vi "多通道并行实测.vi"() -> ()   [LabVIEW 2020]
uses:
  <vilib>/Utility/sysdir.llb/System Directory Type.ctl
  <vilib>/Utility/error.llb/DialogType.ctl
  global/GlobalVariable.vi
  global/SettingVariable.vi
  <vilib>/Analysis/polynomials.llb/Scalar Polynomial Evaluation (DBL).vi
  <vilib>/Analysis/NI_AALPro.lvlib
panel:
  out "T2周期":dbl[](array[numeric]) caption="倍增周期 (s):"
  in  "拟合数":i32(knob)=5 scale=5.0..100.0
  out "多通道并行测量":dbl[][](graph) caption="Waveform Chart - Dark"
  out "四路VO":dbl[](array[numeric]) caption="四路电压输出(V)："
  out "反应性OUT":dbl[](array[numeric])
  out "源与本底开":bool
  in  "源与本底":bool
  out "滤波开":bool
  in  "通量滤波":bool
  out "DRWM开":bool
  in  "动态刻棒":bool
  in  "全量程衔接设置":bool
  in  "添加备注说明":string caption="添加备注说明："
  in  "Start Button":bool
  in  "停止测量":bool
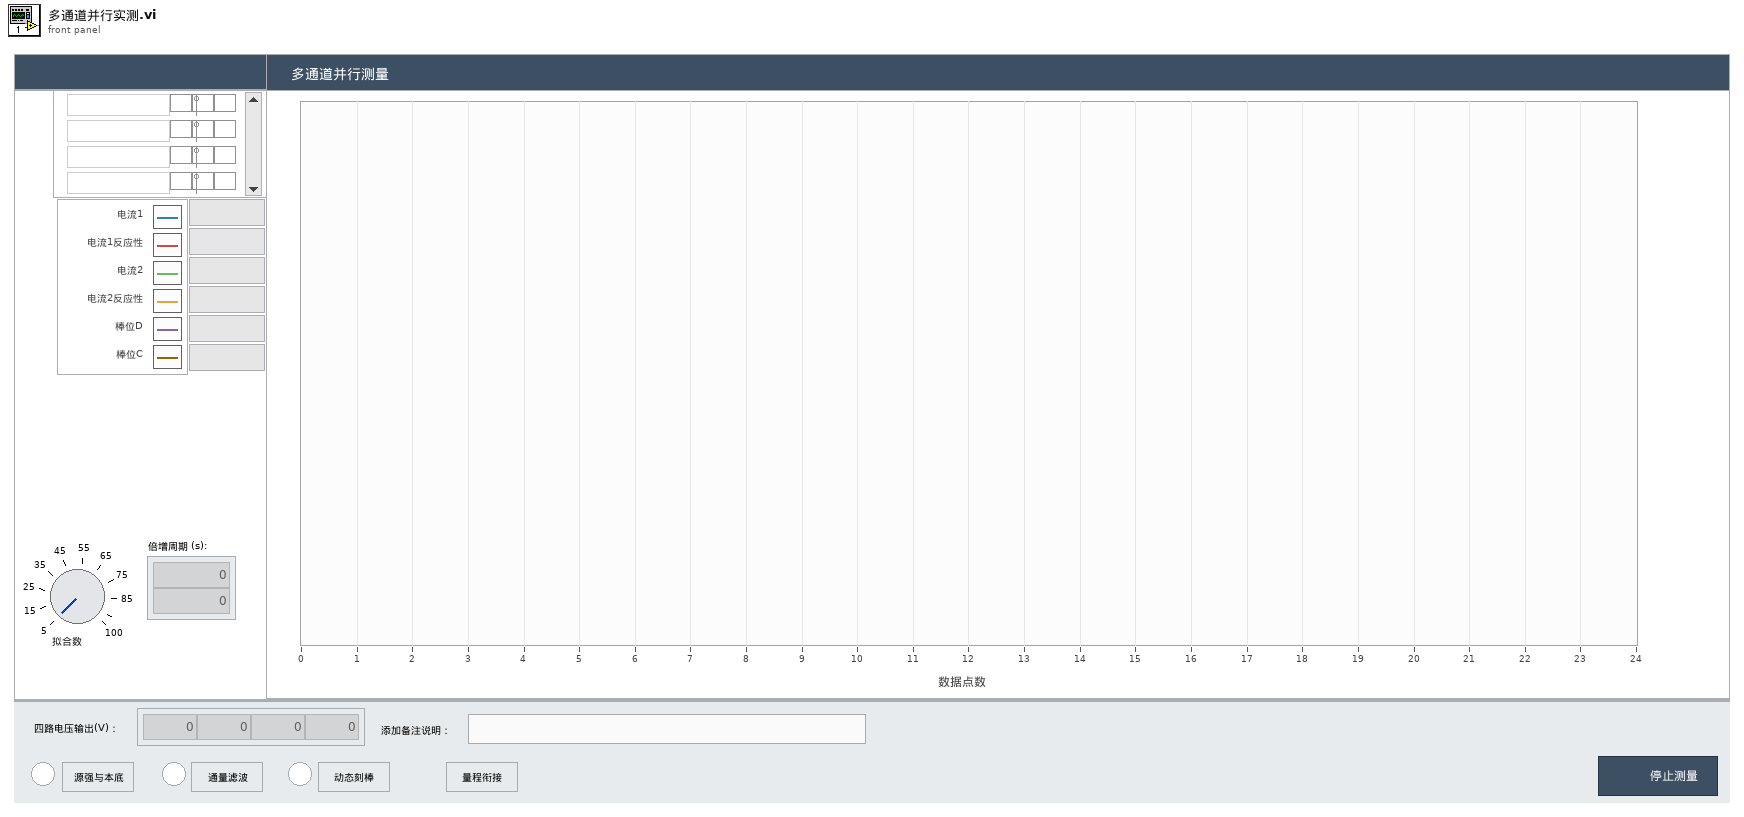
[diagram p1: front panel]
types:
  T1 = enum8{"Enabled", "Disabled", "Disabled and Grayed Out"}
  T2 = enum16{"open", "open or create", "create or replace", "create", "open (read only)"}
  T3 = cluster{"switch":bool, "name":string, "voltage upper":i32, "voltage lower":i32, "physics upper":dbl, "physics lower":dbl, "scale":u16}[]
  T4 = typedef "DialogType.ctl" = u16
  T5 = typedef "System Directory Type.ctl" = i32
  T6 = cluster{"switch":bool, "voltage upper":i32, "voltage lower":i32, "physics upper":dbl, "physics lower":dbl, "input":u16, "log":bool}[]
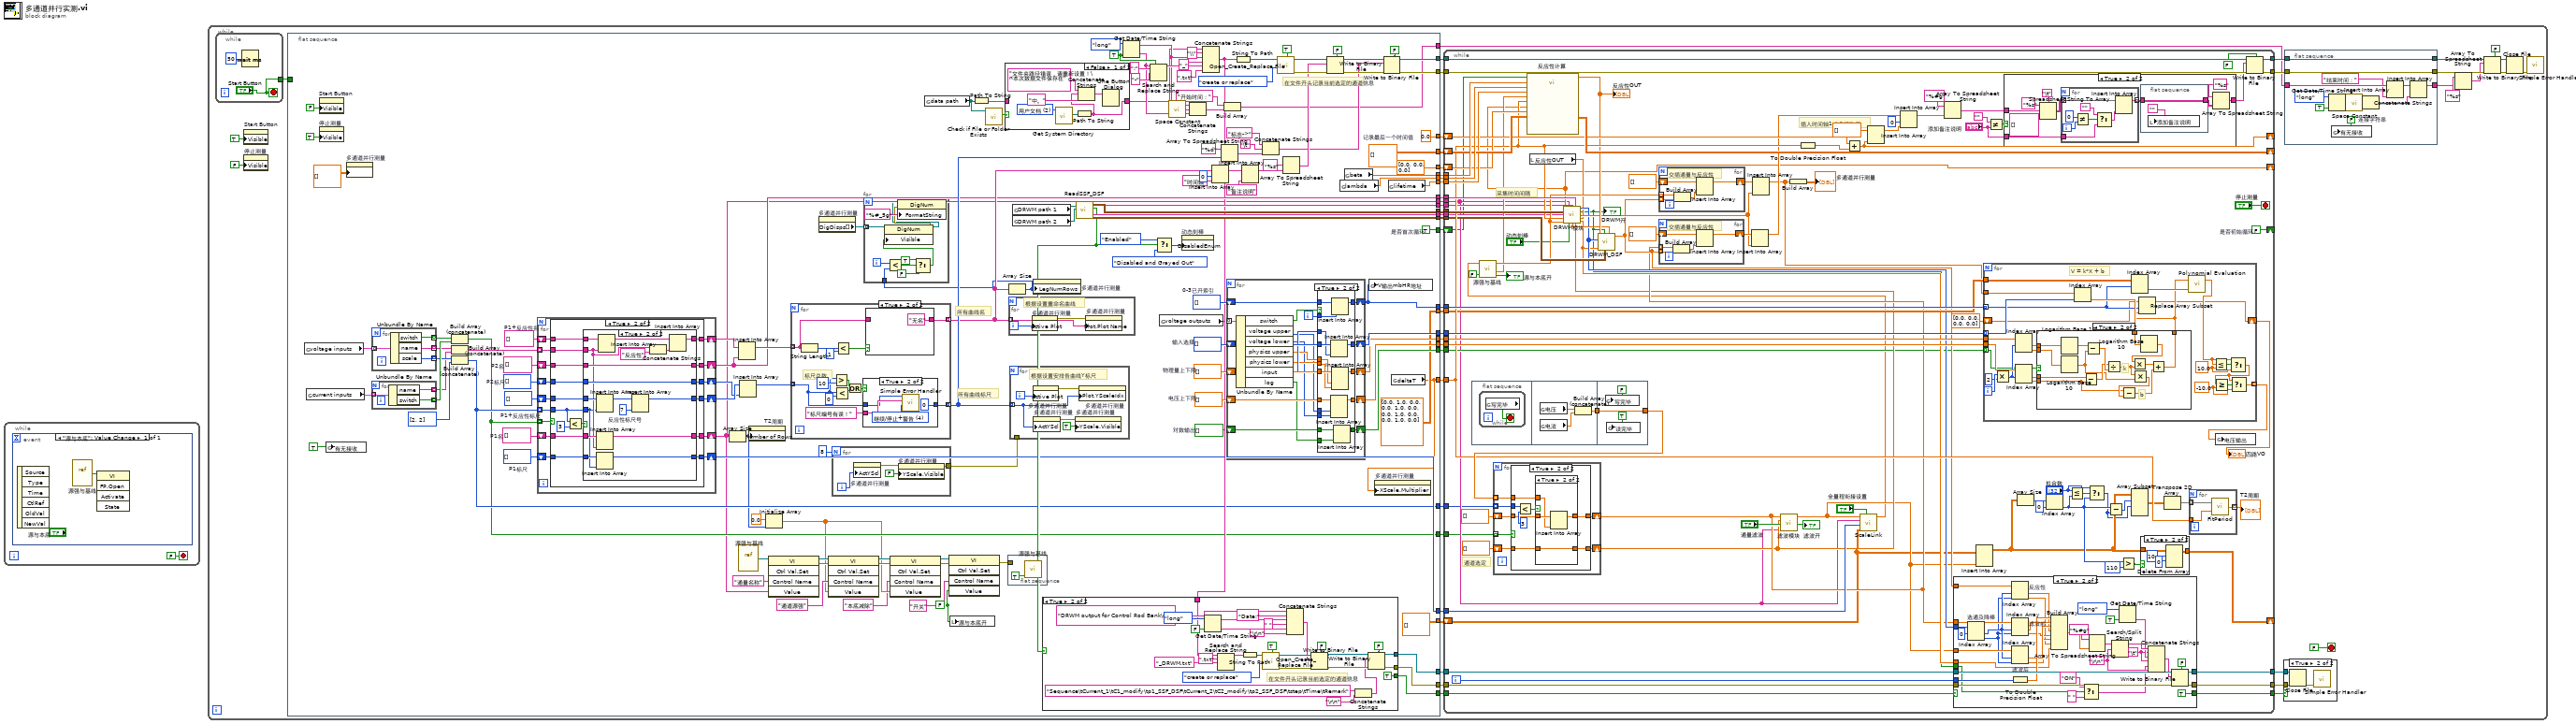
[diagram p0: block diagram]
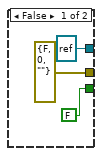
[diagram p4: hidden frame]
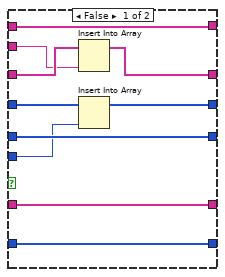
[diagram p8: hidden frame]
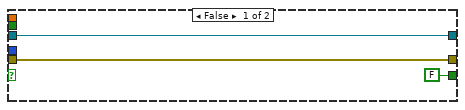
[diagram p10: hidden frame]
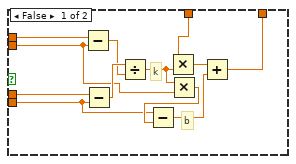
[diagram p12: hidden frame]
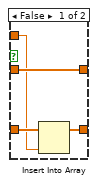
[diagram p15: hidden frame]
diagram:
  n1 = while {
    stop <- FALSE stop-if-true
    n2 = event shown="[0] \"源与本底\": Value Change" {
      selector: _ -> [_]
      dyn-events: _ -> [_]
      timeout: _ -> [_]
      event "源与本底": Value Change {
        n3 = event-data() -> ()  [unwired: 1 in, 6 out]
        n4 = vi-ref "源强与基线.vi"() -> (w2:refnum<vi>)
        n5 = invoke class="VI" method="FP.Open"(reference=w2) -> ()  [unwired: 4 in, 5 out]
      }
    }
  }
  n6 = while {
    stop <- FALSE stop-if-true
    n7 = while {
      tunnel: ["Start Button"] -> w5
      stop <- "Start Button" stop-if-true
      n8 = Wait (ms)(milliseconds to wait=u32 50) -> ()  [unwired: 1 out]
    }
    n9 = property on="Start Button" class="Bool"("Visible"=TRUE) -> ()  [unwired: 2 in, 2 out]
    n10 = property on="停止测量" class="Bool"("Visible"=FALSE) -> ()  [unwired: 2 in, 2 out]
    n11 = flat-sequence {
      tunnel: [sgl[][] [] ("λ*Ci")] -> w50
      tunnel: [w167] -> w47
      tunnel: [w150] -> w46
      tunnel: [w149] -> w45
      tunnel: [w143] -> w44
      tunnel: [sgl[] [0.0, 0.0, 0.0] ("N(0)OUT")] -> w34
      tunnel: [w128] -> w33
      tunnel: [w127] -> w32
      tunnel: [w126] -> w31
      tunnel: [dbl[][] [] ("data")] -> w30
      tunnel: [w122] -> w29
      tunnel: [w114] -> w28
      tunnel: [w113] -> w27
      tunnel: [w112] -> w26
      tunnel: [w111] -> w25
      tunnel: [w110] -> w24
      tunnel: [w109] -> w23
      tunnel: [w107] -> w20
      tunnel: [w104] -> w18
      tunnel: [w103] -> w17
      tunnel: [w102] -> w16
      tunnel: [w101] -> w15
      tunnel: [w98] -> w14
      tunnel: [w67] -> w13
      tunnel: [w86] -> w12
      tunnel: [w85] -> w11
      tunnel: [w84] -> w10
      tunnel: [w72] -> w9
      tunnel: [dbl[][] [[0.0, 1.0, 0.0], [0.0, 1.0, 0.0], [0.0, 1.0, 0.0], [0.0, 1.0, 0.0]]] -> w8
      tunnel: [w78] -> w7
      tunnel: w5 -> [_]
      frame #0 {
        w54 = FALSE
        w87 = i32[] []  # P1标尺
        w88 = string[] []  # P1名
        w105 = bool[] []  # 对数输出
        w124 = i32[] []  # 0-3已开索引
        w129 = sgl[] []  # 电压上下限
        w130 = sgl[] []  # 物理量上下限
        w131 = u16[] []  # 输入选择
        w138 = TRUE ("需要秒？(F)")
        w143 = 0.0  # 记录最后一个时间值
        w163 = string[] []  # P2名
        w162 = i32[] []  # P2标尺
        w164 = i32[] []  # P1+反应性标尺
        w165 = string[] []  # P1+反应性名
        w167 = TRUE  # 是否首次循环
        # "所有曲线标尺"
        # "所有曲线名"
        # "在文件开头记录当前选定的通道信息"
        n12 = global read "SettingVariable.vi" "voltage inputs"() -> (w97:T3)
        n13 = global read "SettingVariable.vi" "current inputs"() -> (w96:cluster{"name":string, "switch":bool}[])
        n14 = property on="Start Button" class="Bool"("Visible"=FALSE) -> ()  [unwired: 2 in, 2 out]
        n15 = property on="停止测量" class="Bool"("Visible"=TRUE) -> ()  [unwired: 2 in, 2 out]
        n16 = global write "GlobalVariable.vi" "有无接收"(TRUE ("写完毕")) -> ()
        n17 = property on="多通道并行测量" class="WFChart (strict)"("History Data"=dbl[][] []) -> ()  [unwired: 2 in, 2 out]
        n18 = for {
          tunnel: w96 -> [w217] mode=indexing
          tunnel: [w216] -> w91 mode=indexing
          tunnel: [w215] -> w94 mode=indexing
          n19 = Unbundle By Name(w217) -> ("name"=w216:string, "switch"=w215:bool)
        }
        n20 = for {
          tunnel: w97 -> [w221] mode=indexing
          tunnel: [w220] -> w95 mode=indexing
          tunnel: [w219] -> w93 mode=indexing
          tunnel: [w218] -> w92 mode=indexing
          n21 = Unbundle By Name(w221) -> ("switch"=w220:bool, "name"=w219:string, "scale"=w218:u16)
        }
        n22 = Build Array (concatenate)(w95, w94) -> (w84:bool[])
        n23 = Build Array (concatenate)(w93, w91) -> (w89:string[])
        n24 = Build Array (concatenate)(w92, u16[] [2, 2] ("array")) -> (w85:u16[])
        n25 = for {
          tunnel: w89 -> [w315] mode=indexing
          shift-right: [w323] -> w161
          shift-left: w165 -> [w322]
          shift-right: [w320] -> w160
          shift-left: w164 -> [w321]
          shift-right: [w318] -> w122
          shift-left: w163 -> [w319]
          shift-right: [w316] -> w159
          shift-left: w162 -> [w317]
          tunnel: w84 -> [w314] mode=indexing
          tunnel: w85 -> [w313] mode=indexing
          shift-right: [w311] -> w67
          shift-left: w88 -> [w312]
          shift-right: [w309] -> w86
          shift-left: w87 -> [w310]
          n26 = case shown="True" w314 {
            tunnel: [w329 w345] -> w323
            tunnel: w322 -> [w329 w341]
            tunnel: w315 -> [_ w340]
            tunnel: [w328 w343] -> w320
            tunnel: w321 -> [w328 w335]
            tunnel: w319 -> [w327 w339]
            tunnel: [w327 w338] -> w318
            tunnel: w317 -> [w326 w337]
            tunnel: [w326 w336] -> w316
            tunnel: w313 -> [_ w334]
            tunnel: w312 -> [w325 w333]
            tunnel: [w325 w332] -> w311
            tunnel: w310 -> [w324 w331]
            tunnel: [w324 w330] -> w309
            frame False {
            }
            frame True {
              n27 = Less?(x=w334, y=3) -> (x < y?=w342:bool)
              n28 = case shown="True" w342 {
                tunnel: w341 -> [w354 w367]
                tunnel: [w354 w372] -> w345
                tunnel: w335 -> [w355 w363]
                tunnel: [w355 w371] -> w343
                tunnel: w340 -> [w351 w360]
                tunnel: w339 -> [w353 w365]
                tunnel: [w352 w365] -> w338
                tunnel: [w348 w364] -> w336
                tunnel: w337 -> [w350 w364]
                tunnel: w334 -> [w349 w356]
                tunnel: w333 -> [w347 w361]
                tunnel: [w347 w359] -> w332
                tunnel: w331 -> [w346 w358]
                tunnel: [w346 w357] -> w330
                frame False {
                  n29 = Insert Into Array(array=w353, new element=w351) -> (w352:string[])  [unwired: 1 in]
                  n30 = Insert Into Array(array=w350, new element=w349) -> (w348:i32[])  [unwired: 1 in]
                }
                frame True {
                  w368 = 7  # 反应性标尺号
                  n31 = Insert Into Array(array=w363, new element=w356) -> (w362:i32[])  [unwired: 1 in]
                  n32 = Insert Into Array(array=w361, new element=w360) -> (w359:string[])  [unwired: 1 in]
                  n33 = Insert Into Array(array=w358, new element=w356) -> (w357:i32[])  [unwired: 1 in]
                  n34 = Insert Into Array(array=w367, new element=w360) -> (w366:string[])  [unwired: 1 in]
                  n35 = Insert Into Array(array=w362, new element=w368) -> (w371:i32[])  [unwired: 1 in]
                  n36 = Concatenate Strings(w360, "反应性" ("字符串")) -> (w369:string)
                  n37 = Insert Into Array(array=w366, new element=w369) -> (w372:string[])  [unwired: 1 in]
                }
              }
            }
          }
        }
        n38 = Array Size(array=w67) -> (size(s)=w66:i32)
        n39 = Insert Into Array(array=w161, new element=w122) -> (w157:string[])  [unwired: 1 in]
        n40 = vi-ref "源强与基线.vi"() -> (w69:refnum<vi>)
        n41 = Insert Into Array(array=w160, new element=w159) -> (w158:i32[])  [unwired: 1 in]
        n42 = property on="T2周期" class="Arr (strict)"("Number of Rows"=w66) -> ()  [unwired: 2 in, 2 out]
        n43 = Initialize Array(0.0 ("element"), w66) -> (w59:dbl[])
        n44 = invoke class="VI" method="Ctrl Val.Set"(reference=w69, "Control Name"="通量名称", "Value"=w67) -> (reference out=w64:refnum<vi>, error out=w63:errorcluster)  [unwired: 2 in, 3 out]
        n45 = for {
          tunnel: w158 -> [w200] mode=indexing
          tunnel: w157 -> [w197] mode=indexing
          tunnel: [w198] -> w148 mode=indexing
          tunnel: [w196] -> w123 mode=indexing
          # "标尺总数"
          n46 = String Length(string=w197) -> (length=w202:i32)
          n47 = Greater?(x=w200, y=10) -> (0:w204:bool)
          n48 = Less?(x=w200, y=0) -> (x < y?=w203:bool)
          n49 = Less?(x=w202, y=1) -> (x < y?=w195:bool)
          n50 = Or(x=w204, y=w203) -> (x .or. y?=w201:bool)
          n51 = case shown="True" w201 {
            tunnel: "标尺编号有误！" ("error source (\" \")") -> [_ w212]
            tunnel: w200 -> [w208 w211]
            tunnel: [w208 0] -> w198
            frame False {
            }
            frame True {
              w210 = T4 4 items=["无对话框", "确定信息", "继续或停止信息", "确定信息＋警告", "继续/停止+警告"] ("type of dialog (OK msg:1)")
              n52 = call <vilib>:"Simple Error Handler.vi"("error code (no error:0)"=w211, "error source (\" \")"=w212, "type of dialog (OK msg:1)"=w210) -> ()  [unwired: 2 in, 5 out]
            }
          }
          n53 = case shown="True" w195 {
            tunnel: w197 -> [w213 _]
            tunnel: [w213 "无名"] -> w196
            frame False {
            }
            frame True {
            }
          }
        }
        n54 = property on="多通道并行测量" class="WFChart (strict)"() -> ("DigDisps[]"=w75:refnum<vi>[])  [unwired: 2 in, 2 out]
        n55 = invoke class="VI" method="Ctrl Val.Set"(reference=w64, error in=w63, "Control Name"="通道源强", "Value"=w59) -> (reference out=w61:refnum<vi>, error out=w60:errorcluster)  [unwired: 1 in, 3 out]
        n56 = for {
          N: 8 -> [_]
          tunnel: [w182] -> w70
          i -> [w181]
          n57 = property on="多通道并行测量" class="WFChart (strict)"("ActYScl"=w181) -> (error out=w183:errorcluster)  [unwired: 2 in, 1 out]
          n58 = property on="多通道并行测量" class="WFChart (strict)"(error in=w183, "YScale.Visible"=FALSE ("Y Scale.Visible")) -> (error out=w182:errorcluster)  [unwired: 1 in, 1 out]
        }
        n59 = invoke class="VI" method="Ctrl Val.Set"(reference=w61, error in=w60, "Control Name"="本底减除", "Value"=w59) -> (reference out=w57:refnum<vi>, error out=w56:errorcluster)  [unwired: 1 in, 3 out]
        n60 = global read "SettingVariable.vi" "data path"() -> (w99:path)
        n61 = invoke class="VI" method="Ctrl Val.Set"(reference=w57, error in=w56, "Control Name"="开关", "Value"=w54) -> (error out=w53:errorcluster)  [unwired: 1 in, 4 out]
        n62 = local write "源与本底开"(w54) -> ()
        n63 = Path To String(path=w99) -> (string=w100:string)
        n64 = call <vilib>:"Check if File or Folder Exists.vi"("path"=w99) -> ("file or folder exists?"=w119:bool)  [unwired: 8 in, 2 out]
        n65 = case shown="False" w119 {
          tunnel: w100 -> [_ w267]
          tunnel: [w262 w267] -> w118
          frame False {
            w266 = T5 2 items=["用户目录"=0, "用户桌面"=1, "用户文档"=2, "用户应用程序数据"=3, "用户设置"=4, "用户临时目录"=5, "公共文档"=6, "公共应用程序数据"=7, "公共设置"=8, "公共缓存"=13, "系统核心库"=9, "系统安装库"=10, "应用程序文件"=11, "启动盘根目录"=12] ("system directory type")
            n66 = call <vilib>:"Get System Directory.vi"("system directory type"=w266) -> ("system directory"=w264:path)  [unwired: 10 in]
            n67 = Path To String(path=w264) -> (string=w262:string)
            n68 = Concatenate Strings("文件夹路径错误，请重新设置！\n本次数据文件保存在" ("消息"), w262, "中。" ("字符串")) -> (w265:string)
            n69 = One Button Dialog(message=w265) -> ()  [unwired: 1 in, 1 out]
          }
          frame True {
          }
        }
        n70 = flat-sequence {
          tunnel: w53 -> [_]
          frame #0 {
            n71 = call "源强与基线.vi"("首次调用？"=TRUE) -> ()  [unwired: 6 in, 3 out]
          }
        }
        n72 = for {
          tunnel: w123 -> [w228] mode=indexing
          i -> [w229]
          # "根据设置重命名曲线"
          n73 = property on="多通道并行测量" class="WFChart (strict)"("Active Plot"=w229) -> (error out=w227:errorcluster)  [unwired: 2 in, 1 out]
          n74 = property on="多通道并行测量" class="WFChart (strict)"(error in=w227, "Plot.Plot Name"=w228) -> ()  [unwired: 1 in, 2 out]
        }
        n75 = Array Size(array=w123) -> (size(s)=w74:i32)
        n76 = for {
          tunnel: w75 -> [w194] mode=indexing
          tunnel: w74 -> [w190]
          i -> [w192]
          n77 = Less?(x=w192, y=w190) -> (x < y?=w191:bool)
          n78 = Select(t=TRUE ("Visible"), s=w191, f=FALSE) -> (s? t:f=w188:bool)
          n79 = property class="DigNum"(reference=w194, "Visible"=w188) -> (reference out=w185:refnum<vi>, error out=w186:errorcluster)  [unwired: 1 in]
          n80 = property class="DigNum"(reference=w185, error in=w186, "FormatString"="%#_5g" ("Format String")) -> ()  [unwired: 2 out]
        }
        n81 = for {
          tunnel: w148 -> [w224] mode=indexing
          tunnel: w70 -> [_]
          i -> [w226]
          # "根据设置安排各曲线Y标尺"
          n82 = property on="多通道并行测量" class="WFChart (strict)"("Active Plot"=w226) -> (error out=w225:errorcluster)  [unwired: 2 in, 1 out]
          n83 = property on="多通道并行测量" class="WFChart (strict)"("ActYScl"=w224) -> (error out=w223:errorcluster)  [unwired: 2 in, 1 out]
          n84 = property on="多通道并行测量" class="WFChart (strict)"(error in=w223, "YScale.Visible"=TRUE ("Y Scale.Visible")) -> ()  [unwired: 1 in, 2 out]
          n85 = property on="多通道并行测量" class="WFChart (strict)"(error in=w225, "Plot.YScaleIdx"=w224) -> ()  [unwired: 1 in, 2 out]
        }
        n86 = global read "SettingVariable.vi" "DRWM path 1"() -> (w80:path)
        n87 = global read "SettingVariable.vi" "DRWM path 2"() -> (w79:path)
        n88 = property on="多通道并行测量" class="WFChart (strict)"("LegNumRows"=w74) -> ()  [unwired: 2 in, 2 out]
        n89 = call "ReadSSF_DSF.vi"("DRWM path 2"=w79, "DRWM path 1"=w80) -> ("DSF"=w113:cluster{"x":dbl, "y":dbl}[][], "因子棒号"=w112:string[], "SF_0K"=w106:bool, "SSF"=w114:cluster{"x":dbl, "y":dbl}[][], "文件INFO"=w111:string)  [unwired: 5 in]
        n90 = Get Date/Time String(date format (0)=enum16{"short", "long", "abbreviated"}."long" ("日期格式(0)"), want seconds? (F)=w138) -> (date string=w136:string, time string=w135:string)  [unwired: 1 in]
        n91 = Search and Replace String(replace all?=w138, input string=w135, search string=":", replace string="-" ("replace string (\"\")")) -> (result string=w174:string)  [unwired: 4 in, 3 out]
        n92 = Select(t=T1."Enabled" ("禁用"), s=w106, f=T1."Disabled and Grayed Out" ("禁用")) -> (s? t:f=w117:T1)
        n93 = global read "SettingVariable.vi" "voltage outputs"() -> (w81:T6)
        n94 = call <vilib>:"Space Constant.vi"() -> ("String"=w137:string)
        n95 = property on="动态刻棒" class="Bool"("DisabledEnum"=w117) -> ()  [unwired: 2 in, 2 out]
        n96 = Concatenate Strings ("连接字符串")(w136, w137, w135) -> (w134:string)
        n97 = Concatenate Strings ("连接字符串")(w118, "\\" ("字符串"), w136, "_" ("string"), w174, ".txt" ("string")) -> (w108:string)
        n98 = case shown="True" w106 {
          tunnel: [refnum<file> refnum ("refnum out") w243] -> w110
          tunnel: [errorcluster {"status"=FALSE, "code"=0, "source"=""} ("error out") w242] -> w109
          tunnel: w108 -> [_ w241]
          tunnel: [FALSE ("预置数组或字符串大小？(T)") TRUE ("预置数组或字符串大小？(T)")] -> w107
          frame False {
          }
          frame True {
            # "在文件开头记录当前选定的通道信息"
            n99 = Get Date/Time String(date format (0)=enum16{"short", "long", "abbreviated"}."long" ("日期格式(0)"), want seconds? (F)=FALSE ("需要秒？(F)")) -> (date string=w247:string, time string=w245:string)  [unwired: 1 in]
            n100 = Search and Replace String(input string=w241, search string=".txt" ("搜索字符串"), replace string="_DRWM.txt" ("字符串")) -> (result string=w238:string)  [unwired: 5 in, 3 out]
            n101 = String To Path(string=w238) -> (path=w253:path)
            n102 = call <vilib>:"Open_Create_Replace File.vi"("advisory dialog? (display:T)"=TRUE, "function (open:0)"=T2."create or replace", "file path"=w253) -> ("error out"=w260:errorcluster, "refnum"=w258:refnum<file>)  [unwired: 5 in, 2 out]
            n103 = Concatenate Strings("DRWM output for Control Rod Bank\n" ("连接的字符串"), "Date:" ("字符串"), w247, " " ("字符串"), w245, "\r\n") -> (w244:string)
            n104 = Write to Binary File(file (use dialog)=w258, data=w244, error in=w260, 5:FALSE ("预置数组或字符串大小？(T)")) -> (refnum out=w255:refnum<file>, error out=w254:errorcluster)  [unwired: 2 in, 1 out]
            n105 = Concatenate Strings("Sequence\tCurrent_1\tC1_modify\tρ1_SSF_DSF\tCurrent_2\tC2_modify\tρ2_SSF_DSF\tstep\tTime\tRemark" ("连接的字符串"), "\r\n") -> (w235:string)
            n106 = Write to Binary File(file (use dialog)=w255, data=w235, error in=w254, 5:FALSE ("预置数组或字符串大小？(T)")) -> (refnum out=w243:refnum<file>, error out=w242:errorcluster)  [unwired: 2 in, 1 out]
          }
        }
        n107 = Insert Into Array(array=w123, index=0 ("索引"), new element="时间轴" ("新元素/子数组")) -> (w142:string[])
        n108 = Array To Spreadsheet String(array=w148, 3:"%d" ("format string")) -> (spreadsheet string=w147:string)  [unwired: 1 in]
        n109 = Build Array("开始时间：" ("字符串"), w134) -> (w98:string[])
        n110 = for {
          shift-right: [w285] -> w128
          shift-left: w131 -> [w286]
          shift-right: [w281] -> w127
          shift-left: w130 -> [w282]
          shift-right: [w283] -> w126
          shift-left: w129 -> [w284]
          shift-right: [w279] -> w78
          shift-left: w124 -> [w280]
          shift-right: [w276] -> w104
          shift-left: w105 -> [w277]
          tunnel: w81 -> [w275] mode=indexing
          i -> [w278]
          n111 = Unbundle By Name(w275) -> ("switch"=w274:bool, "voltage upper"=w270:i32, "voltage lower"=w269:i32, "physics upper"=w272:dbl, "physics lower"=w271:dbl, "input"=w273:u16, "log"=w268:bool)
          n112 = case shown="True" w274 {
            tunnel: w286 -> [w291 w308]
            tunnel: [w291 w307] -> w285
            tunnel: w273 -> [_ w306]
            tunnel: w284 -> [w289 w305]
            tunnel: [w289 w304] -> w283
            tunnel: w282 -> [w290 w303]
            tunnel: [w290 w302] -> w281
            tunnel: w272 -> [_ w301]
            tunnel: w271 -> [_ w300]
            tunnel: w270 -> [_ w299]
            tunnel: w269 -> [_ w298]
            tunnel: w280 -> [w288 w297]
            tunnel: w278 -> [_ w296]
            tunnel: [w288 w295] -> w279
            tunnel: w268 -> [_ w294]
            tunnel: w277 -> [w287 w293]
            tunnel: [w287 w292] -> w276
            frame False {
            }
            frame True {
              n113 = Insert Into Array(array=w308, new element=w306) -> (w307:u16[])  [unwired: 1 in]
              n114 = Insert Into Array(array=w305, new element #1=w299, new element #2=w298) -> (w304:sgl[])  [unwired: 1 in]
              n115 = Insert Into Array(array=w297, new element=w296) -> (w295:i32[])  [unwired: 1 in]
              n116 = Insert Into Array(array=w303, new element #1=w301, new element #2=w300) -> (w302:sgl[])  [unwired: 1 in]
              n117 = Insert Into Array(array=w293, new element=w294) -> (w292:bool[])  [unwired: 1 in]
            }
          }
        }
        n118 = String To Path(string=w108) -> (path=w120:path)
        n119 = Insert Into Array(array=w142, new element="备注说明" ("新元素/子数组")) -> (w141:string[])  [unwired: 1 in]
        n120 = Concatenate Strings("标志->" ("字符串"), "\t", w147) -> (w144:string)
        n121 = call <vilib>:"Open_Create_Replace File.vi"("advisory dialog? (display:T)"=TRUE, "function (open:0)"=T2."create or replace", "file path"=w120) -> ("error out"=w172:errorcluster, "refnum"=w169:refnum<file>)  [unwired: 5 in, 2 out]
        n122 = Array To Spreadsheet String(array=w141, 3:"%s" ("format string")) -> (spreadsheet string=w166:string)  [unwired: 1 in]
        n123 = Write to Binary File(file (use dialog)=w169, data=w166, error in=w172, 5:FALSE ("预置数组或字符串大小？(T)")) -> (refnum out=w152:refnum<file>, error out=w151:errorcluster)  [unwired: 2 in, 1 out]
        n124 = global read "SettingVariable.vi" "lambda"() -> (w101:dbl[])
        n125 = global read "SettingVariable.vi" "beta"() -> (w102:dbl[])
        n126 = global write "GlobalVariable.vi" "V输出mbHR地址"(w78) -> ()
        n127 = Write to Binary File(file (use dialog)=w152, data=w144, error in=w151, 5:FALSE ("预置数组或字符串大小？(T)")) -> (refnum out=w150:refnum<file>, error out=w149:errorcluster)  [unwired: 2 in, 1 out]
        n128 = global read "SettingVariable.vi" "lifetime"() -> (w103:dbl)
        n129 = global read "SettingVariable.vi" "deltaT"() -> (w72:dbl)
        n130 = property on="多通道并行测量" class="WFChart (strict)"("XScale.Multiplier"=w72) -> ()  [unwired: 2 in, 2 out]
      }
    }
    n131 = while {
      shift-right: [w481] -> _
      shift-left: w50 -> [w482]
      tunnel: w16 -> [w483]
      tunnel: w15 -> [w488]
      tunnel: w17 -> [w480]
      shift-right: [w487] -> _
      shift-left: w47 -> [w390]
      tunnel: w46 -> [w479]
      tunnel: w45 -> [w486]
      tunnel: [w485] -> w49
      tunnel: w9 -> [w443]
      tunnel: [w478] -> w48
      shift-right: [w468] -> _
      shift-left: w44 -> [w471]
      shift-right: [w398] -> _
      shift-left: w34 -> [w461]
      shift-right: [w452] -> _
      shift-left: w30 -> [w410]
      tunnel: w33 -> [w456]
      tunnel: w32 -> [w455]
      tunnel: w31 -> [w454]
      tunnel: w7 -> [w453]
      tunnel: w12 -> [w448]
      tunnel: w28 -> [w446]
      tunnel: w27 -> [w441]
      tunnel: w29 -> [w447]
      tunnel: w13 -> [w397]
      tunnel: w8 -> [w434]
      tunnel: w26 -> [w431]
      tunnel: w25 -> [w430]
      tunnel: w24 -> [w429]
      tunnel: w23 -> [w428]
      tunnel: [w427] -> w22
      tunnel: [w426] -> w21
      tunnel: w20 -> [w420]
      tunnel: [w419] -> w19
      tunnel: w18 -> [w406]
      tunnel: w11 -> [w395]
      tunnel: w10 -> [w396]
      i -> [w423]
      stop <- "停止测量" stop-if-true
      w487 = FALSE  # 是否初始循环
      # "通道选定"
      # "插入时间轴1或多行数据"
      # "采集时间间隔"
      n132 = flat-sequence {
        tunnel: [w490] -> w414
        tunnel: [w494] -> w473
        tunnel: w414 -> [w494]
        frame #0 {
          n133 = while {
            stop <- w489 stop-if-true
            n134 = global read "GlobalVariable.vi" "写完毕"() -> (w489:bool)
          }
        }
        frame #1 {
          n135 = global read "GlobalVariable.vi" "电压"() -> (w492:dbl[])
          n136 = global read "GlobalVariable.vi" "电流"() -> (w491:dbl[])
          n137 = Build Array (concatenate)(w492, w491) -> (w490:dbl[])
        }
        frame #2 {
          n138 = global write "GlobalVariable.vi" "写完毕"(FALSE ("写完毕")) -> ()
          n139 = global write "GlobalVariable.vi" "读完毕"(TRUE ("写完毕")) -> ()
        }
      }
      n140 = for {
        shift-right: [w627] -> w413
        shift-left: dbl[] [] ("data") -> [w628]
        shift-right: [w625] -> w412
        shift-left: dbl[] [] ("data") -> [w626]
        tunnel: w473 -> [w624] mode=indexing
        tunnel: w396 -> [w623] mode=indexing
        tunnel: w395 -> [w622] mode=indexing
        n141 = case shown="True" w623 {
          tunnel: w622 -> [_ w637]
          tunnel: w628 -> [w630 w635]
          tunnel: [w630 w634] -> w627
          tunnel: w626 -> [w629 w633]
          tunnel: [w629 w632] -> w625
          tunnel: w624 -> [_ w631]
          frame False {
          }
          frame True {
            n142 = Less?(x=w637, y=3) -> (x < y?=w636:bool)
            n143 = case shown="True" w636 {
              tunnel: w635 -> [w640 w645]
              tunnel: [w640 w644] -> w634
              tunnel: w633 -> [w642 w646]
              tunnel: [w641 w646] -> w632
              tunnel: w631 -> [w639 w643]
              frame False {
                n144 = Insert Into Array(array=w642, new element=w639) -> (w641:dbl[])  [unwired: 1 in]
              }
              frame True {
                n145 = Insert Into Array(array=w645, new element=w643) -> (w644:dbl[])  [unwired: 1 in]
              }
            }
          }
        }
      }
      n146 = local read "反应性OUT"() -> (w417:dbl[])
      n147 = call "滤波模块.vi"("通量名称"=w397, "执行:调用时显示前面板"="通量滤波", "P2信号"=w412, "通量in"=w413) -> ("滤波开"=→"滤波开":bool, "通量out"=w411:dbl[])  [unwired: 5 in, 1 out]
      n148 = To Double Precision Float(number=w443) -> (double precision float=w407:dbl)
      n149 = Add(x=w471, y=w407) -> (x+y=w468:dbl)
      n150 = call "ScaleLink.vi"("执行:调用时显示前面板"="全量程衔接设置", "曲线输入"=w410, "通量标尺"=w448, "通量名称"=w397, "通量输入"=w411) -> ("通量输出"=w392:dbl[])  [unwired: 6 in]
      n151 = call "源强与基线.vi"("首次调用？"=FALSE, "通量in"=w392) -> ("源与基线灯"=→"源与本底开":bool, "源强out"=w432:dbl[], "通量out"=w437:dbl[])  [unwired: 5 in]
      n152 = call "DRWM模块.vi"("通量名称"=w397, "因子说明"=w430, "P2名称"=w447, "SSF因子"=w446, "因子棒名"=w431, "时间步长"=w443, "反应性in"=w417, "通量in"=w437, "执行:调用时显示前面板"="动态刻棒", "P2信号"=w412) -> ("通量out"=w398:dbl[], "上下段通量索引"=w425:u16[], "DRWM开"=w415:bool, "P2信号out"=w436:dbl[], "棒限"=w433:dbl[], "动态棒位"=w418:dbl)
      "DRWM开" <- w415
      n153 = call "反应性计算.vi"("首循环？"=w390, "λi*Ci(0)"=w482, "N(0)IN"=w461, "βi"=w483, "λi"=w488, "中子寿命"=w480, "源强"=w432, "采集间隔"=w443, "中子注量率"=w398) -> ("λi*Ci(t)"=w481:sgl[][], "反应性OUT"=w442:dbl[])  [unwired: 5 in]
      "反应性OUT" <- w442
      n154 = call "DRWM_DSF.vi"("棒限值"=w433, "DSF因子"=w441, "DRWM开"=w415, "动态棒位"=w418, "上下段通量选择"=w425, "反应性in"=w442) -> ("反应性out"=w424:dbl[])  [unwired: 5 in]
      n155 = for {
        tunnel: w413 -> [w537] mode=indexing
        tunnel: w424 -> [w536] mode=indexing
        shift-right: [w538] -> w438
        shift-left: dbl[] [] ("平滑掉数据") -> [w539]
        # "交插通量与反应性"
        n156 = Build Array(w537, w536) -> (w535:dbl[])
        n157 = Insert Into Array(array=w539, new element=w535) -> (w538:dbl[])  [unwired: 1 in]
      }
      n158 = for {
        tunnel: w437 -> [w649] mode=indexing
        tunnel: w424 -> [w648] mode=indexing
        shift-right: [w650] -> w472
        shift-left: dbl[] [] ("平滑掉数据") -> [w651]
        # "交插通量与反应性"
        n159 = Build Array(w649, w648) -> (w647:dbl[])
        n160 = Insert Into Array(array=w651, new element=w647) -> (w650:dbl[])  [unwired: 1 in]
      }
      n161 = Insert Into Array(array=w438, new element=w436) -> (w435:dbl[])  [unwired: 1 in]
      n162 = Insert Into Array ("数组插入")(array=w472, new element=w436) -> (w408:dbl[])  [unwired: 1 in]
      n163 = Build Array(w408) -> (→"多通道并行测量":dbl[][])
      n164 = Insert Into Array(array=dbl[] [], new element=w468) -> (w469:dbl[])  [unwired: 1 in]
      n165 = Insert Into Array(array=w435, index=0 ("索引 (行)"), new element=w469) -> (w409:dbl[])
      n166 = Array To Spreadsheet String(array=w409, 3:"%#g" ("format string")) -> (spreadsheet string=w463:string)  [unwired: 1 in]
      n167 = case shown="True" w420 {
        tunnel: w429 -> [w498 w533]
        tunnel: w428 -> [w497 w532]
        tunnel: [w498 w531] -> w427
        tunnel: [w497 w530] -> w426
        tunnel: w425 -> [_ w528]
        tunnel: w413 -> [_ w526]
        tunnel: w411 -> [_ w525]
        tunnel: w424 -> [_ w524]
        tunnel: w423 -> [_ w521]
        tunnel: [FALSE ("预置数组或字符串大小？(T)") TRUE ("预置数组或字符串大小？(T)")] -> w419
        tunnel: w418 -> [_ w499]
        tunnel: w415 -> [_ w505]
        frame False {
        }
        frame True {
          w504 = "\r\n"
          w503 = "\t"
          n168 = Index Array "选通及降棒"(array=w528, index #1=0 ("索引")) -> (element #1=w523:u16, element #2=w522:u16)  [unwired: 1 in]
          n169 = Index Array "反应性"(array=w524, index #1=w523, index #2=w522) -> (element #1=w517:dbl, element #2=w514:dbl)
          n170 = Index Array "滤波前"(array=w526, index #1=w523, index #2=w522) -> (element #1=w519:dbl, element #2=w516:dbl)
          n171 = Index Array "滤波后"(array=w525, index #1=w523, index #2=w522) -> (element #1=w518:dbl, element #2=w515:dbl)
          n172 = To Double Precision Float(number=w521) -> (double precision float=w520:dbl)
          n173 = Build Array(w520, w519, w518, w517, w516, w515, w514, w499) -> (w513:dbl[])
          n174 = Select(t="ON" ("format string"), s=w505, f=" " ("format string")) -> (s? t:f=w502:string)
          n175 = Array To Spreadsheet String(array=w513, 3:"%#g" ("format string")) -> (spreadsheet string=w511:string)  [unwired: 1 in]
          n176 = Search/Split String(string=w511, search string/char (-)=w504) -> (substring before match=w512:string)  [unwired: 1 in, 2 out]
          n177 = Get Date/Time String(date format (0)=enum16{"short", "long", "abbreviated"}."long" ("日期格式(0)"), want seconds? (F)=TRUE ("需要秒？(F)")) -> (time string=w507:string)  [unwired: 1 in, 1 out]
          n178 = Concatenate Strings(w512, w503, w507, w503, w502, w504) -> (w510:string)
          n179 = Write to Binary File(file (use dialog)=w533, data=w510, error in=w532, 5:FALSE ("预置数组或字符串大小？(T)")) -> (refnum out=w531:refnum<file>, error out=w530:errorcluster)  [unwired: 2 in, 1 out]
        }
      }
      n180 = Insert Into Array(array=w410, new element=w411) -> (w421:dbl[][])  [unwired: 2 in]
      n181 = for {
        tunnel: w456 -> [w564] mode=indexing
        tunnel: w455 -> [w570]
        tunnel: w454 -> [w569]
        tunnel: w408 -> [w565]
        tunnel: w453 -> [w548] mode=indexing
        tunnel: w434 -> [w554]
        tunnel: w406 -> [w549] mode=indexing
        tunnel: [w550] -> w405 mode=indexing
        shift-right: [w545] -> w393
        shift-left: dbl[] [0.0, 0.0, 0.0, 0.0] ("四路VO") -> [w547]
        i -> [w568]
        w556 = sgl -10.0 ("y")
        w558 = sgl 10.0 ("y")
        # "V = k*X + b"
        n182 = Multiply(x=w568, y=2) -> (x*y=w566:i32)
        n183 = Index Array(array=w570, index #1=w566) -> (element #1=w563:sgl, element #2=w560:sgl)  [unwired: 1 in]
        n184 = Index Array(array=w569, index #1=w566) -> (element #1=w561:sgl, element #2=w552:sgl)  [unwired: 1 in]
        n185 = Index Array(array=w565, index=w564) -> (element=w562:dbl)
        n186 = case shown="True" w549 {
          tunnel: w563 -> [w582 w591]
          tunnel: w562 -> [w579 w585]
          tunnel: w561 -> [w578 w587]
          tunnel: w560 -> [w576 w590]
          tunnel: w552 -> [w572 w586]
          tunnel: [w571 w583] -> w546
          frame False {
            # "b"
            # "k"
            n187 = Subtract(x=w582, y=w576) -> (x-y=w580:sgl)
            n188 = Subtract(x=w578, y=w572) -> (x-y=w581:sgl)
            n189 = Divide(x=w581, y=w580) -> (x/y=w577:sgl)
            n190 = Multiply(x=w579, y=w577) -> (x*y=w574:dbl)
            n191 = Multiply(x=w577, y=w576) -> (x*y=w575:sgl)
            n192 = Subtract(x=w572, y=w575) -> (x-y=w573:sgl)
            n193 = Add(x=w574, y=w573) -> (x+y=w571:dbl)
          }
          frame True {
            # "b"
            # "k"
            n194 = Logarithm Base 10(1:w591) -> (0:w589:sgl)
            n195 = Logarithm Base 10(1:w590) -> (0:w588:sgl)
            n196 = Subtract(x=w587, y=w586) -> (x-y=w592:sgl)
            n197 = Subtract(x=w589, y=w588) -> (x-y=w593:sgl)
            n198 = Divide(x=w592, y=w593) -> (x/y=w594:sgl)
            n199 = Multiply(x=w594, y=w588) -> (x*y=w595:sgl)
            n200 = Subtract(x=w586, y=w595) -> (x-y=w597:sgl)
            n201 = Logarithm Base 10(1:w585) -> (0:w584:dbl)
            n202 = Multiply(x=w584, y=w594) -> (x*y=w596:dbl)
            n203 = Add(x=w596, y=w597) -> (x+y=w583:dbl)
          }
        }
        n204 = Index Array(array=w554, index (row)=w548) -> (element=w553:dbl[])  [unwired: 1 in]
        n205 = Replace Array Subset(array=w547, new element=w546, index=w548) -> (w545:dbl[])
        n206 = call-poly <vilib>:"Polynomial Evaluation.vi"("P(x)"=w553, "a"=w546) -> ("P(a)"=w551:dbl)  [unwired: 1 out]
        n207 = Less Or Equal?(x=w551, y=w558) -> (x <= y?=w559:bool)
        n208 = Select(t=w551, s=w559, f=w558) -> (s? t:f=w555:dbl)
        n209 = Greater Or Equal?(x=w555, y=w556) -> (x >= y?=w557:bool)
        n210 = Select(t=w555, s=w557, f=w556) -> (s? t:f=w550:dbl)
      }
      "四路VO" <- w393
      n211 = Not Equal?(x="", y="添加备注说明") -> (x != y?=w464:bool)
      n212 = case shown="True" w464 {
        tunnel: [w601 w602] -> w462
        tunnel: "添加备注说明" -> [_ w611]
        tunnel: w463 -> [w601 w606]
        frame False {
        }
        frame True {
          n213 = Spreadsheet String To Array(delimiter (Tab)="\t", format string="%s", spreadsheet string=w606, array type (2D Dbl)=string[][] [] ("添加的数组")) -> (array=w607:string[][])
          n214 = for {
            tunnel: w607 -> [w621] mode=indexing
            tunnel: [w620] -> w605 mode=indexing
            tunnel: w611 -> [w615]
            i -> [w619]
            n215 = Not Equal?(x=0 ("y"), y=w619) -> (x != y?=w617:bool)
            n216 = Select(t="", s=w617, f=w615) -> (s? t:f=w616:string)
            n217 = Insert Into Array(array=w621, new element=w616) -> (w620:string[])  [unwired: 1 in]
          }
          n218 = flat-sequence {
            tunnel: w605 -> [w612]
            tunnel: [w612] -> w603
            frame #0 {
              n219 = local write "添加备注说明"("") -> ()
            }
          }
          n220 = Array To Spreadsheet String(array=w603, 3:"%s" ("format string")) -> (spreadsheet string=w602:string)  [unwired: 1 in]
        }
      }
      n221 = Array Size(array=w421) -> (size(s)=w460:i32[])
      n222 = Index Array(array=w460, index=0 ("索引")) -> (element=w422:i32)
      n223 = Less Or Equal?(x="拟合数", y=w422) -> (x <= y?=w458:bool)
      n224 = Select(t="拟合数", s=w458, f=w422) -> (s? t:f=w403:i32)
      n225 = Subtract(x=w422, y=w403) -> (x-y=w404:i32)
      n226 = Greater?(x=w422, y=110) -> (0:w450:bool)
      n227 = Array Subset ("数组子集")(array=w421, index (row)=w404, length (row)=w403) -> (w401:dbl[][])  [unwired: 2 in]
      n228 = case shown="True" w450 {
        tunnel: w421 -> [w540 w544]
        tunnel: [w540 w543] -> w452
        frame False {
        }
        frame True {
          n229 = Delete From Array ("删除数组元素")(array=w544, length=10 ("y"), index (row)=0 ("索引 (行)")) -> (array with subset deleted=w543:dbl[][])  [unwired: 1 in, 1 out]
        }
      }
      n230 = Transpose 2D Array(2D array=w401) -> (transposed array=w402:dbl[][])
      n231 = for {
        tunnel: w402 -> [w600] mode=indexing
        tunnel: [w598] -> w399 mode=indexing
        tunnel: w443 -> [w599]
        n232 = call "FitPeriod.vi"("delta"=w599, "curve"=w600) -> ("T2"=w598:dbl)
      }
      "T2周期" <- w399
      n233 = global write "GlobalVariable.vi" "电压输出"(w405) -> ()
      n234 = Write to Binary File(file (use dialog)=w479, data=w462, error in=w486, 5:FALSE ("预置数组或字符串大小？(T)")) -> (refnum out=w478:refnum<file>, error out=w485:errorcluster)  [unwired: 2 in, 1 out]
    }
    n235 = case shown="True" w19 {
      tunnel: w22 -> [_ w374]
      tunnel: w21 -> [_ w373]
      frame False {
      }
      frame True {
        n236 = Close File(refnum=w374, error in=w373) -> (error out=w375:errorcluster)  [unwired: 1 out]
        n237 = call <vilib>:"Simple Error Handler.vi"("error in (no error)"=w375) -> ()  [unwired: 4 in, 5 out]
      }
    }
    n238 = flat-sequence {
      tunnel: w49 -> [w382]
      tunnel: w48 -> [w383]
      tunnel: w14 -> [w381]
      tunnel: [w383] -> w38
      tunnel: [w382] -> w37
      tunnel: [w377] -> w41
      frame #0 {
        n239 = Get Date/Time String(date format (0)=enum16{"short", "long", "abbreviated"}."long" ("日期格式(0)"), want seconds? (F)=TRUE ("需要秒？(F)")) -> (date string=w386:string, time string=w385:string)  [unwired: 1 in]
        n240 = global write "GlobalVariable.vi" "有无接收"(FALSE ("写完毕")) -> ()
        n241 = call <vilib>:"Space Constant.vi"() -> ("String"=w384:string)
        n242 = Concatenate Strings "连接字符串"(w386, w384, w385) -> (w378:string)
        n243 = Insert Into Array(array=w381, new element="结束时间：" ("字符串")) -> (w379:string[])  [unwired: 1 in]
        n244 = Insert Into Array(array=w379, new element=w378) -> (w377:string[])  [unwired: 1 in]
      }
    }
    n245 = Array To Spreadsheet String(array=w41, 3:"%s" ("format string")) -> (spreadsheet string=w36:string)  [unwired: 1 in]
    n246 = Write to Binary File(file (use dialog)=w38, data=w36, error in=w37, 5:FALSE ("预置数组或字符串大小？(T)")) -> (refnum out=w40:refnum<file>, error out=w39:errorcluster)  [unwired: 2 in, 1 out]
    n247 = Close File(refnum=w40, error in=w39) -> (error out=w43:errorcluster)  [unwired: 1 out]
    n248 = call <vilib>:"Simple Error Handler.vi"("error in (no error)"=w43) -> ()  [unwired: 4 in, 5 out]
  }
